vi "Configure Channels.vi"(8 "error in":errorcluster, 11 "DO DAQmx Fixed Freq PWM CFG in":refnum<class "DO DAQmx Fixed Freq PWM CFG.lvclass">) -> (0 "error out":errorcluster, 3 "DO DAQmx Fixed Freq PWM CFG out":refnum<class "DO DAQmx Fixed Freq PWM CFG.lvclass">)   [LabVIEW 2023, in "DO DAQmx Fixed Freq PWM CFG.lvclass"]
uses:
  DO DAQmx Fixed Freq PWM CFG.lvclass
  D:/git/HAL/HAL/Configurations/CFG JSON/CFG JSON.lvclass
  D:/git/HAL/HAL GOOP4/DAQmx/DAQmx Base CFG/DAQmx Base CFG.lvclass
  D:/git/HAL/HAL/Configurations/CFG Base/CFG Base.lvclass
  DAQmx Base CFG/DAQmx Base CFG.lvclass/DAQmx Base CFG.ctl
  Configurations/CFG Base/CFG Base.lvclass/CFG Base.ctl
  DO DAQmx Fixed Freq PWM CFG.lvclass/DO DAQmx Fixed Freq PWM CFG.ctl
  6411cd84-0cc3-40a4-b609-a223cd4ed0c4.vi
  <vilib>/JDP Science/JSONtext/Find Item.vi
  <vilib>/JDP Science/JSONtext/Next JSON Value.vi
  <vilib>/JDP Science/JSONtext/String Subset.vi
  <vilib>/JDP Science/JSONtext/Parsing/Advance past next JSON Value (inlined COPY).vi
  <vilib>/JDP Science/JSONtext/Parsing/Advance past whitespace.vi
  <vilib>/JDP Science/JSONtext/Parsing/Advance past String.vi
  <vilib>/JDP Science/JSONtext/Parsing/Advance past Number.vi
  <vilib>/JDP Science/JSONtext/Parsing/Advance past Line Ending.vi
  <vilib>/JDP Science/JSONtext/Parsing/Parse Full Path or Item Name.vi
  <vilib>/JDP Science/JSONtext/Parsing/Advance past Array.vi
  <vilib>/JDP Science/JSONtext/Parsing/Advance past Object.vi
  <vilib>/JDP Science/JSONtext/support/Error Cluster From Code.vi
  <vilib>/JDP Science/JSONtext/Offset/Find Item Locations by Path.vi
  <vilib>/JDP Science/JSONtext/JSON text to Variant.vi
  <vilib>/Utility/error.llb/Error Cluster From Error Code.vi
  <vilib>/DAQmx/create/channels.llb/DAQmx Create Channel (DO-Digital Output).vi
  <vilib>/JDP Science/JSONtext/LVClass Serializer/JSONtext LVClass Serializer.lvclass
  <vilib>/ErrorRing/Error Ring.xnode
  DAQmx Base CFG/DAQmx Base CFG.lvclass
  <resource>/objmgr/daqmx.rc
  Configurations/CFG JSON/CFG JSON.lvclass
  Configurations/CFG Base/CFG Base.lvclass
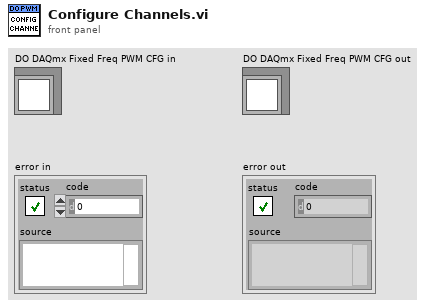
[diagram p1: front panel]
types:
  T1 = cluster{"Name":string, "Enabled":bool, "Frequency":dbl, "Duty Cycle":dbl, "Invert Lines":bool, "Line Grouping":string}[]
  T2 = enum16{"one channel for each line", "one channel for all lines"}
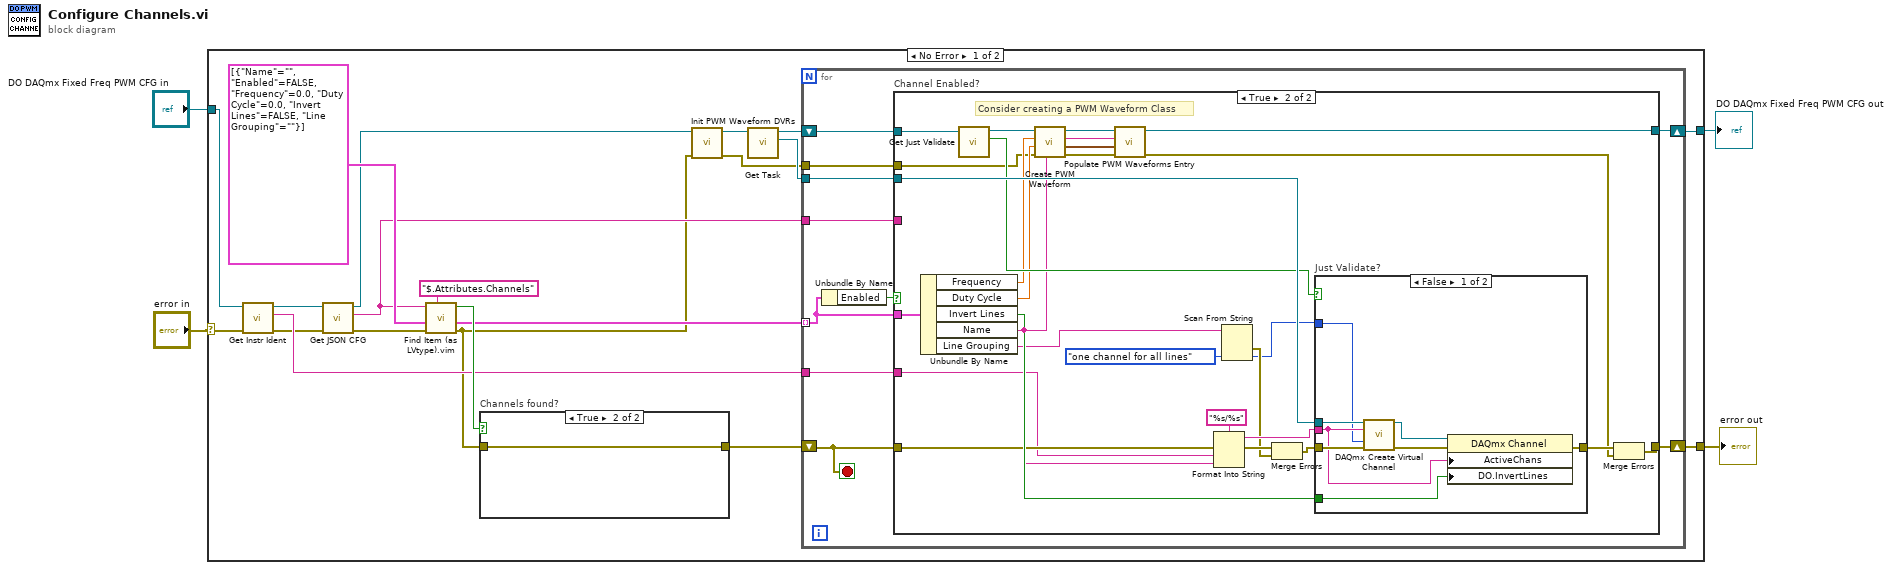
[diagram p0: block diagram]
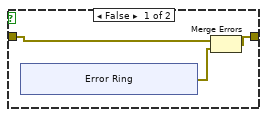
[diagram p2: hidden frame]
diagram:
  n1 = case shown="No Error" "error in" {
    selector: "error in" -> [w17 w82]
    tunnel: "DO DAQmx Fixed Freq PWM CFG in" -> [w13 w83]
    tunnel: [w18 w82] -> w2
    tunnel: [w12 w83] -> w1
    frame No Error {
      n2 = call-dynamic "Get Instr Ident.vi"("error in"=w17, "CFG JSON in"=w13) -> ("error out"=w5:errorcluster, "Instr Ident"=w19:string, "CFG JSON out"=w20:refnum<class "DO DAQmx Fixed Freq PWM CFG.lvclass">)  [unwired: 7 in]
      n3 = call "Get JSON CFG.vi"("CFG JSON in"=w20) -> ("<JSON> CFG"=w16:string, "CFG JSON out"=w8:refnum<class "DO DAQmx Fixed Freq PWM CFG.lvclass">)  [unwired: 9 in]
      n4 = call "Find Item (as LVtype).vim"("$Path or Item Name"="$.Attributes.Channels", "error in (no error)"=w5, "Data Type and Default Value"=T1 [{"Name"="", "Enabled"=FALSE, "Frequency"=0.0, "Duty Cycle"=0.0, "Invert Lines"=FALSE, "Line Grouping"=""}], "JSON"=w16) -> ("error out"=w7:errorcluster, "Data"=w14:T1, "Found"=w22:bool)  [unwired: 4 in, 1 out]
      n5 = case "Channels found?" shown="True" w22 {
        tunnel: w7 -> [w26 w32]
        tunnel: [w24 w32] -> w10
        frame False {
          n6 = xnode "Error Ring"() -> ("error out"=w25:errorcluster)
          n7 = Merge Errors(w26, w25) -> (w24:errorcluster)
        }
        frame True {
        }
      }
      n8 = call "Init PWM Waveform DVRs.vi"("error in"=w7, "DO DAQmx Fixed Freq PWM CFG in"=w8) -> ("error out"=w6:errorcluster, "DO DAQmx Fixed Freq PWM CFG out"=w9:refnum<class "DO DAQmx Fixed Freq PWM CFG.lvclass">)  [unwired: 8 in]
      n9 = call "Get Task.vi"("DAQmx Base CFG in"=w9) -> ("Task"=w15:refnum<k21>, "DAQmx Base CFG out"=w11:refnum<class "DO DAQmx Fixed Freq PWM CFG.lvclass">)  [unwired: 9 in]
      n10 = for {
        tunnel: w14 -> [w39] mode=indexing
        shift-right: [w42] -> w18
        shift-left: w10 -> [w41]
        tunnel: w19 -> [w40]
        tunnel: w16 -> [w38]
        tunnel: w15 -> [w37]
        shift-right: [w36] -> w12
        shift-left: w11 -> [w35]
        tunnel: w6 -> [w34]
        stop <- w41 stop-if-true
        n11 = Unbundle By Name(w39) -> ("Enabled"=w33:bool)
        n12 = case "Channel Enabled?" shown="True" w33 {
          tunnel: [w44 w69] -> w42
          tunnel: w41 -> [w44 w60]
          tunnel: w40 -> [_ w59]
          tunnel: w39 -> [_ w72]
          tunnel: [w43 w49] -> w36
          tunnel: w38 -> [_ _]
          tunnel: w37 -> [_ w67]
          tunnel: w35 -> [w43 w66]
          tunnel: w34 -> [_ w52]
          frame False {
          }
          frame True {
            # "Consider creating a PWM Waveform Class"
            n13 = Unbundle By Name(w72) -> ("Frequency"=w63:dbl, "Duty Cycle"=w62:dbl, "Invert Lines"=w70:bool, "Name"=w54:string, "Line Grouping"=w48:string)
            n14 = call "Get Just Validate.vi"("CFG Base in"=w66) -> ("Just Validate"=w64:bool, "CFG Base out"=w65:refnum<class "DO DAQmx Fixed Freq PWM CFG.lvclass">)  [unwired: 9 in]
            n15 = call-dynamic "Create PWM Waveform.vi"("Channel Ident"=w54, "error in"=w52, "Duty Cycle"=w62, "Frequency"=w63, "DO DAQmx Fixed Freq PWM CFG in"=w65) -> ("error out"=w56:errorcluster, "PWM Waveform"=w50:digitalwaveform, "Channel Ident out"=w51:string, "DO DAQmx Fixed Freq PWM CFG out"=w55:refnum<class "DO DAQmx Fixed Freq PWM CFG.lvclass">)  [unwired: 3 in]
            n16 = call "Populate PWM Waveforms Entry.vi"("error in"=w56, "PWM Waveform"=w50, "Channel Ident"=w51, "DO DAQmx Fixed Freq PWM CFG in"=w55) -> ("error out"=w68:errorcluster, "DO DAQmx Fixed Freq PWM CFG in 2"=w49:refnum<class "DO DAQmx Fixed Freq PWM CFG.lvclass">)  [unwired: 6 in]
            n17 = Format Into String(format string="%s/%s", error in=w60, w59, w54) -> (resulting string=w57:string, error out=w58:errorcluster)  [unwired: 1 in]
            n18 = Scan From String(input string=w48, default 1=T2."one channel for all lines" ("Line Grouping")) -> (error out=w47:errorcluster, output 1=w46:T2)  [unwired: 3 in, 2 out]
            n19 = Merge Errors(w58, w47) -> (w53:errorcluster)
            n20 = case "Just Validate?" shown="False" w64 {
              tunnel: w53 -> [w80 w81]
              tunnel: w57 -> [w74 _]
              tunnel: w67 -> [w79 _]
              tunnel: [w77 w81] -> w71
              tunnel: w70 -> [w75 _]
              tunnel: w46 -> [w73 _]
              frame False {
                n21 = call-poly <vilib>:"DAQmx Create Virtual Channel.vi"("task in"=w79, "lines"=w74, "line grouping"=w73, "error in"=w80) -> ("task out"=w76:refnum<k21>, "error out"=w78:errorcluster)  [unwired: 10 in]
                n22 = property class="DAQmx Channel"(reference=w76, error in=w78, "ActiveChans"=w74, "DO.InvertLines"=w75) -> (error out=w77:errorcluster)  [unwired: 1 out]
              }
              frame True {
              }
            }
            n23 = Merge Errors(w71, w68) -> (w69:errorcluster)
          }
        }
      }
    }
    frame Error {
    }
  }
  "error out" <- w2
  "DO DAQmx Fixed Freq PWM CFG out" <- w1
